vi "SelectGraph.vi"(10 "reference":refnum<vi>, 11 "Array in":refnum<vi>) -> ()   [LabVIEW 2018]
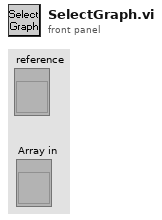
[diagram p1: front panel]
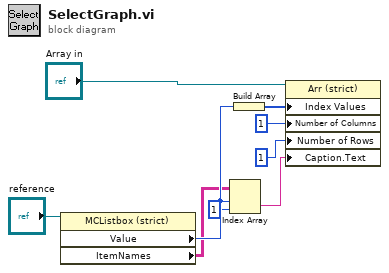
[diagram p0: block diagram]
diagram:
  n1 = property on="Property Node" class="MCListbox (strict)"(reference="reference") -> ("Value"=w5:i32, "ItemNames"=w4:string[][])  [unwired: 1 in, 2 out]
  n2 = Index Array(array=w4, index (row)=w5, index (col)=1 ("disabled index (col)")) -> (element=w2:string)
  n3 = Build Array(w5) -> (w9:i32[])
  n4 = property on="Property Node" class="Arr (strict)"(reference="Array in", "Index Values"=w9, "Number of Columns"=u32 1 ("millisecond multiple"), "Number of Rows"=u32 1 ("millisecond multiple"), "Caption.Text"=w2) -> ()  [unwired: 1 in, 2 out]
